vi "Pack and Send TCP Message.vi"(8 "error in (no error)":errorcluster, 10 "Tcp Message":T1={"Command"="", "Data"=[], "Script ID"=0, "LabVIEW Server ID"="zxcvbnm,", "Python Message ID"=0}, 11 "TCP Network Connection in":refnum<k5>) -> (0 "error out":errorcluster, 3 "TCP Network Connection out":refnum<k5>, 4 "Message Length":i32)   [LabVIEW 2013, in "TS.lvlib"]
doc: "This VI packages up the TCP Message, which is of the type TS.lvlib:LabVIEW Python Connector Message.ctl (our fundamental data type) into a string like this: Command|Script ID|[\"First String\", \"Second String\"]. This gets JSONed into a single string and sent over the connection. Make sure you don't include any pipes in your command or your data pieces!"
uses:
  TS.lvlib
  LabVIEW Python Connector Message.ctl
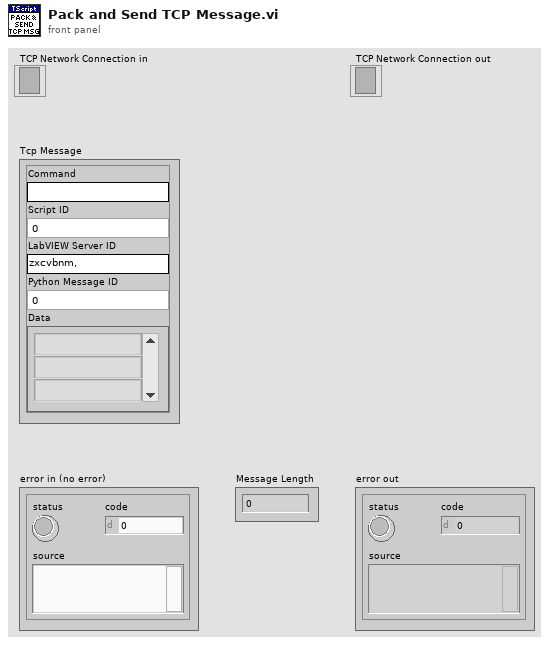
[diagram p1: front panel]
types:
  T1 = typedef "TS.lvlib/LabVIEW Python Connector Message.ctl" = cluster{"Command":string, "Data":string[], "Script ID":i64, "LabVIEW Server ID":string, "Python Message ID":i32}
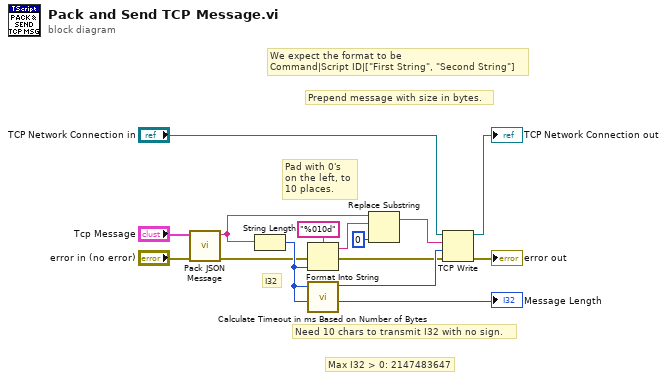
[diagram p0: block diagram]
diagram:
  # "Pad with 0's\non the left, to\n10 places."
  # "Max I32 > 0: 2147483647"
  # "Need 10 chars to transmit I32 with no sign."
  # "I32"
  # "Prepend message with size in bytes."
  # "We expect the format to be\nCommand|Script ID|[\"First String\", \"Second String\"]"
  n1 = call "Pack JSON Message.vi"("error in (no error)"="error in (no error)", "Tcp Message"="Tcp Message") -> ("error out"=w2:errorcluster, "String"=w7:string)  [unwired: 8 in]
  n2 = String Length(string=w7) -> (length=w4:i32)
  "Message Length" <- w4
  n3 = Format Into String(format string="%010d", error in=w2, w4) -> (resulting string=w3:string, error out=w1:errorcluster)  [unwired: 1 in]
  n4 = call "Calculate Timeout in ms Based on Number of Bytes.vi"("Number of Bytes"=w4) -> ("Timeout (ms)"=w10:i32)  [unwired: 10 in]
  n5 = Replace Substring(2:0 ("length (len. of substring)"), 4:w3, 5:w7) -> (1:w6:string)  [unwired: 1 in, 1 out]
  n6 = TCP Write(connection ID="TCP Network Connection in", data in=w6, error in (no error)=w1, 9:w10) -> (connection ID out=→"TCP Network Connection out":refnum<k5>, error out=→"error out":errorcluster)  [unwired: 1 out]
